vi "RSZVB Get User Connector.vi"(8 "error in (no error)":errorcluster {"code" format="%.0x"}, 9 "Port (1)":i32=1, 10 "Channel (1)":i32=1, 11 "VISA session":refnum<visa-resource-name>) -> (0 "error out":errorcluster {"code" format="%.0x"}, 1 "Connector":string, 2 "Connector Gender":i32, 3 "dup VISA session":refnum<visa-resource-name>)   [LabVIEW 2011]
doc: "This VI retuns a user-defined connector type at a specified port <Port> and its gender.\n\nRemote-control command(s):\n[SENSe<Ch>:]CORRection:COLLect:SCONnection<port_no>?"
uses:
  _utility/RSZVB Global Data.vi
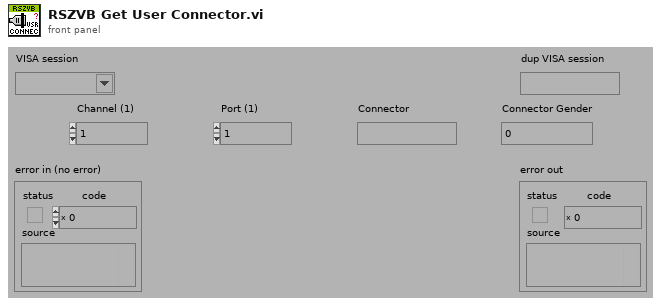
[diagram p1: front panel]
types:
  T1 = cluster{"Error Checking (T: On)":bool, "Installed Options":string[], "Data Valid?":bool, "Ports":i32, "Model":string[], "Option Checking (T: On)":bool}[]
  T2 = cluster{"Error Checking (T: On)":bool, "Installed Options":string[], "Data Valid?":bool, "Ports":i32, "Model":string[], "Option Checking (T: On)":bool}
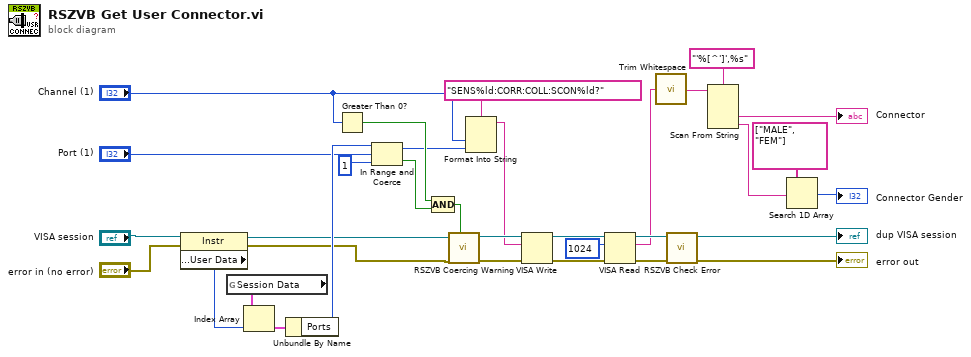
[diagram p0: block diagram]
diagram:
  n1 = property class="Instr"(reference="VISA session", error in="error in (no error)") -> (reference out=w1:refnum<visa-resource-name>, error out=w2:errorcluster, "General Settings:User Data"=w23:u32)
  n2 = global read "RSZVB Global Data.vi" "Session Data"() -> (w24:T1)
  n3 = Index Array(array=w24, index=w23) -> (element=w25:T2)
  n4 = Unbundle By Name(w25) -> ("Ports"=w22:i32)
  n5 = Greater Than 0?(x="Channel (1)") -> (x > 0?=w26:bool)
  n6 = In Range and Coerce(upper limit=w22, x="Port (1)", lower limit=1) -> (coerced(x)=w21:i32, In Range?=w29:bool)
  n7 = Compound Arithmetic op=AND(w26, w29) -> (w28:bool)
  n8 = call "RSZVB Coercing Warning.vi"("In Range?"=w28, "error in (no error)"=w2, "VISA session"=w1) -> ("error out"=w30:errorcluster, "dup VISA session"=w31:refnum<visa-resource-name>)  [unwired: 7 in]
  n9 = Format Into String(format string="SENS%ld:CORR:COLL:SCON%ld?", "Channel (1)", w21) -> (resulting string=w27:string)  [unwired: 2 in, 1 out]
  n10 = VISA Write(VISA resource name=w31, write buffer=w27, error in (no error)=w30) -> (VISA resource name out=w3:refnum<visa-resource-name>, error out=w4:errorcluster)  [unwired: 1 out]
  n11 = VISA Read(VISA resource name=w3, byte count=u32 1024 ("byte count (0)"), error in (no error)=w4) -> (VISA resource name out=w15:refnum<visa-resource-name>, read buffer=w13:string, error out=w14:errorcluster)  [unwired: 1 out]
  n12 = call <vilib>:"Trim Whitespace.vi"("string"=w13) -> ("trimmed string"=w11:string)  [unwired: 1 in]
  n13 = call "RSZVB Check Error.vi"("error in (no error)"=w14, "VISA session"=w15) -> ("error out"=→"error out":errorcluster, "dup VISA session"=→"dup VISA session":refnum<visa-resource-name>)  [unwired: 8 in]
  n14 = Scan From String(format string="'%[^']',%s", input string=w11) -> (output 1=→"Connector":string, output 2=w6:string)  [unwired: 4 in, 3 out]
  n15 = Search 1D Array(1D array=string[] ["MALE", "FEM"] ("array 2"), element=w6) -> (index of element=→"Connector Gender":i32)  [unwired: 1 in]
